vi "Write Data.vi"(10 "数据":i32, 11 "硬件任务消息输入":refnum<class "硬件任务消息.lvclass">) -> (3 "硬件任务消息输出":refnum<class "硬件任务消息.lvclass">)   [LabVIEW 2015, in "硬件操作者.lvlib" / "硬件任务消息.lvclass"]
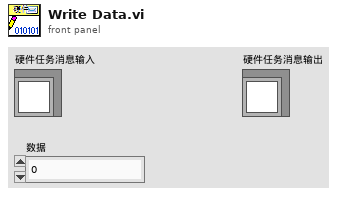
[diagram p1: front panel]
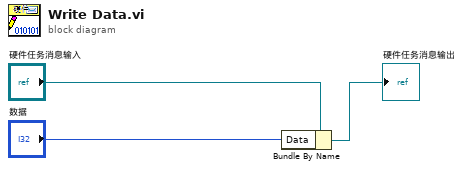
[diagram p0: block diagram]
diagram:
  n1 = Bundle By Name(cluster="硬件任务消息输入", "Data"="数据") -> (→"硬件任务消息输出":refnum<class "硬件任务消息.lvclass">)
